vi "niRFSTS SG Load Waveforms.vi"(0 "Semiconductor Module Context":T1, 5 "Waveform File Names":string[](array[string]), 7 "Sequence Path":path, 9 "Port":string) -> (15 "Error Out":errorcluster)   [LabVIEW 2014]
uses:
  <vilib>/NI_TestStand_SemiconductorModule/NI_TestStand_Semiconductor_Module.lvlibp/PinMap/General/SemiconductorModuleContext.ctl
  <vilib>/NI_TestStand_SemiconductorModule/NI_TestStand_Semiconductor_Module.lvlibp/PinMap/RF/RFSG/PinToNIRFSGSessions.vi
  <instrlib>/niRFSGPlayback/niRFSGPlayback Read Waveform From File (1 Wfm,TDMS, CDB).vi
  <instrlib>/niRFSGPlayback/niRFSGPlayback Read and Download Waveform From File (1 Wfm, 1 RFSG, TDMS).vi
  <vilib>/NI_TestStand_SemiconductorModule/NI_TestStand_Semiconductor_Module.lvlibp
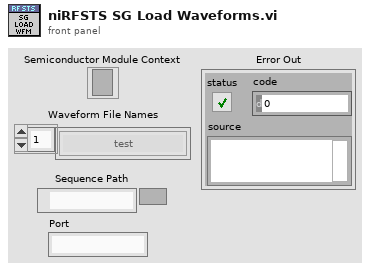
[diagram p1: front panel]
types:
  T1 = typedef "NI_TestStand_Semiconductor_Module.lvlibp/SemiconductorModuleContext.ctl" = refnum<k7>
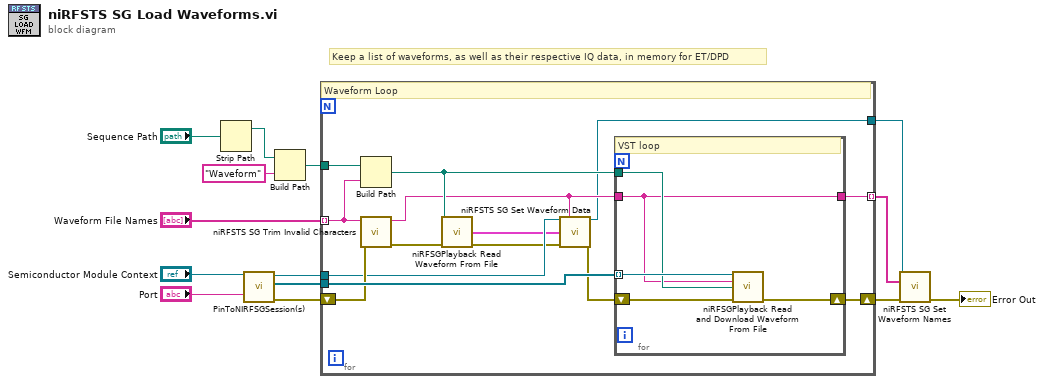
[diagram p0: block diagram]
diagram:
  # "Keep a list of waveforms, as well as their respective IQ data, in memory for ET/DPD"
  n1 = Strip Path(path="Sequence Path") -> (stripped path=w2:path)  [unwired: 1 out]
  n2 = call-poly <vilib>:"PinToNIRFSGSession(s).vi"("Pin"="Port", "Semiconductor Module Context"="Semiconductor Module Context") -> ("error out"=w7:errorcluster, "Instrument Sessions"=w8:refnum<k15>[], "Semiconductor Module Context Out"=w9:T1)  [unwired: 6 in, 1 out]
  n3 = Build Path(base path=w2, name or relative path="Waveform") -> (appended path=w1:path)
  n4 = for {
    tunnel: "Waveform File Names" -> [w27] mode=indexing
    tunnel: w8 -> [w28]
    shift-right: [w25] -> w13
    shift-left: w7 -> [w26]
    tunnel: w9 -> [w24]
    tunnel: [w17] -> w11
    tunnel: [w16] -> w10 mode=indexing
    tunnel: w1 -> [w15]
    # "Waveform Loop"
    n5 = Build Path(base path=w15, name or relative path=w27) -> (appended path=w21:path)
    n6 = call "niRFSTS SG Trim Invalid Characters.vi"("error in (no error)"=w26, "Waveform Name In"=w27) -> ("error out"=w19:errorcluster, "Waveform Name Out"=w20:string)  [unwired: 8 in]
    n7 = call-poly <instrlib>:"niRFSGPlayback Read Waveform From File.vi"("file path"=w21, "error in"=w19) -> ("waveform out"=w18:cluster{"t0":dbl, "dt":dbl, "y":cdb[]}, "error out"=w22:errorcluster)  [unwired: 12 in]
    n8 = call "niRFSTS SG Set Waveform Data.vi"("TSM Context in"=w24, "Waveform Name"=w20, "Waveform"=w18, "error in (no error)"=w22) -> ("TSM Context out"=w17:T1, "error out"=w23:errorcluster)  [unwired: 10 in]
    n9 = for {
      shift-right: [w32] -> w25
      shift-left: w23 -> [w31]
      tunnel: w20 -> [w29]
      tunnel: w28 -> [w33] mode=indexing
      tunnel: w21 -> [w30]
      tunnel: [w29] -> w16
      # "VST loop"
      n10 = call-poly <instrlib>:"niRFSGPlayback Read and Download Waveform From File.vi"("instrument handle in"=w33, "waveform name"=w29, "file path"=w30, "error in"=w31) -> ("error out"=w32:errorcluster)  [unwired: 10 in, 1 out]
    }
  }
  n11 = call "niRFSTS SG Set Waveform Names.vi"("TSM Context in"=w11, "Waveform Names"=w10, "error in (no error)"=w13) -> ("error out"=→"Error Out":errorcluster)  [unwired: 11 in, 1 out]
